vi "Read Status.vi"() -> (0 "Status Data":T1)   [LabVIEW 2012]
doc: "The Basic Serial Read and Write example performs a Serial Port Read, a Serial Port Write, or a combination of these actions. The user selects the actions (read or write) on the front panel. If both are selected, the VI will write the data first, read data, and then close the VISA session that is opened to the port. This VI will wait until the specified number of bytes is received at the port or until a termination character is read.\n\nINSTRUCTIONS:\n1) Select the serial resource and configuration parameters (baud rate, data bits, parity, stop bits, flow control).\n2) Select the operations to be performed. \n3) Connect the serial port to your device. If no device is available, perform a loopback test by doing one of the following. Short pins 2 and 3 on a RS-232 cable or short pin 4 to pin 8 and pin 5 to pin 9 on a RS-485/422 cable. \n4) Run the VI to see the data read. (The \"read string\" will match the \"string to write\" if a loopback test was performed.)\n\nNote: The parameters set for the serial port must match the parameters of the connected instrument or device. In this example, the bytes to read parameter specifies the number of bytes that the serial port reads. If there were more bytes at the port than the number specified in bytes to read, those bytes would not be read. Also, if you specify to read more bytes than the number of bytes actually read, you might receive a timeout error message.\n\nOn the block diagram, the Configure Serial Port VI sets the configuration parameters. The front panel displays the controls used to configure the basic parameters, such as baud rate, data bits, and parity. Constants configure the other parameters the user probably does not need set. After the VISA Configure Serial Port VI opens the VISA session and configures the port, the VI passes the VISA resource name to other VIs that perform operations on that VISA resource. The VISA Write function sends a command to the serial device and the VISA Read function returns data based on the command. The VISA Close function then closes the reference to the serial device. It is important to close the reference; otherwise communication through with that port through protocols other than VISA might not be possible."
uses:
  Correlator port.vi
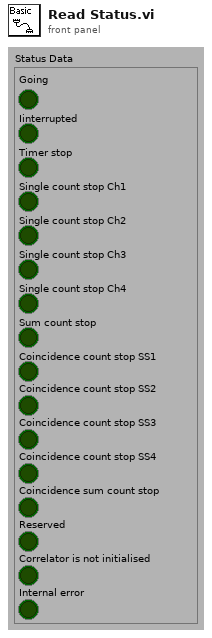
[diagram p1: front panel]
types:
  T1 = cluster{"Going":bool, "Iinterrupted":bool, "Timer stop":bool, "Single count stop Ch1":bool, "Single count stop Ch2":bool, "Single count stop Ch3":bool, "Single count stop Ch4":bool, "Sum count stop":bool, "Coincidence count stop SS1":bool, "Coincidence count stop SS2":bool, "Coincidence count stop SS3":bool, "Coincidence count stop SS4":bool, "Coincidence sum count stop":bool, "Reserved":bool, "Correlator is not initialised":bool, "Internal error":bool}
  T2 = cluster{"unsigned byte array[0]":u8, "unsigned byte array[1]":u8}
  T3 = cluster{"Boolean array[0]":bool, "Boolean array[1]":bool, "Boolean array[2]":bool, "Boolean array[3]":bool, "Boolean array[4]":bool, "Boolean array[5]":bool, "Boolean array[6]":bool, "Boolean array[7]":bool}
  T4 = cluster{"Boolean array[0]":bool, "Boolean array[1]":bool, "Boolean array[2]":bool, "Boolean array[3]":bool, "Boolean array[4]":bool, "Boolean array[5]":bool, "Boolean array[6]":bool, "Boolean array[7]":bool, "Boolean array[0]":bool, "Boolean array[1]":bool, "Boolean array[2]":bool, "Boolean array[3]":bool, "Boolean array[4]":bool, "Boolean array[5]":bool, "Boolean array[6]":bool, "Boolean array[7]":bool}
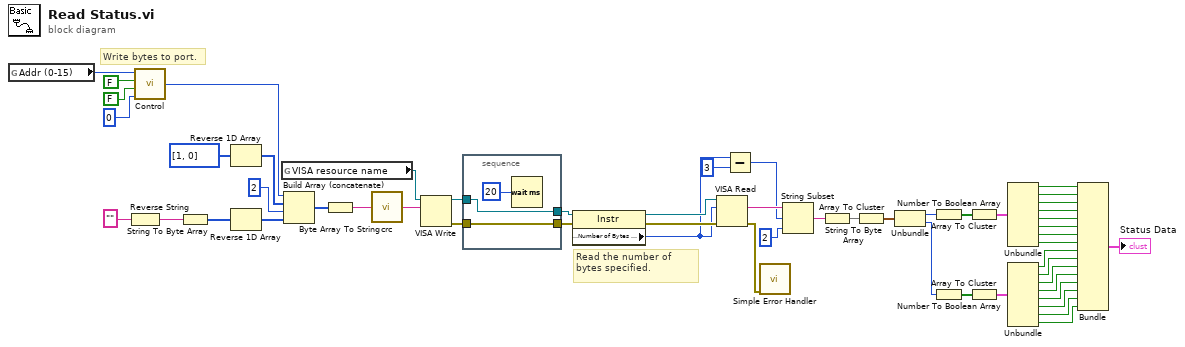
[diagram p0: block diagram]
diagram:
  # "Read the number of bytes specified."
  # "Write bytes to port."
  n1 = global read "Correlator port.vi" "Addr (0-15)"() -> (w7:i8)
  n2 = Reverse String(1:"" ("Data")) -> (0:w9:string)
  n3 = call "Control.vi"("Page"=i8 0, "Error"=FALSE, "Write"=FALSE, "Addr"=w7) -> ("Control Byte"=w19:u32)
  n4 = String To Byte Array(string=w9) -> (unsigned byte array=w14:u8[])
  n5 = Reverse 1D Array(array=i8[] [1, 0] ("Offset")) -> (reversed array=w17:i8[])
  n6 = Reverse 1D Array(array=w14) -> (reversed array=w13:u8[])
  n7 = global read "Correlator port.vi" "VISA resource name"() -> (w8:refnum<visa-resource-name>)
  n8 = Build Array (concatenate)(w19, w17, u8 2 ("Length"), w13) -> (w12:u32[])
  n9 = Byte Array To String(unsigned byte array=w12) -> (string=w11:string)
  n10 = call "crc.vi"("Input string"=w11) -> ("Output (with crc)"=w10:string)
  n11 = VISA Write(VISA resource name=w8, write buffer=w10) -> (VISA resource name out=w52:refnum<visa-resource-name>, error out=w54:errorcluster)  [unwired: 1 in, 1 out]
  n12 = stacked-sequence {
    tunnel: w54 -> [w57]
    tunnel: [w57] -> w53
    tunnel: w52 -> [w56]
    tunnel: [w56] -> w51
    frame #0 {
      n13 = Wait (ms)(milliseconds to wait=u32 20 ("delay before read (ms)")) -> ()  [unwired: 1 out]
    }
  }
  n14 = property class="Instr"(reference=w51, error in=w53) -> (reference out=w5:refnum<visa-resource-name>, error out=w4:errorcluster, "Serial Settings:Number of Bytes at Serial Port"=w3:u32)
  n15 = VISA Read(VISA resource name=w5, byte count=w3, error in (no error)=w4) -> (read buffer=w50:string, error out=w6:errorcluster)  [unwired: 2 out]
  n16 = Subtract(x=w3, y=u32 3) -> (x-y=w1:u32)
  n17 = call <vilib>:"Simple Error Handler.vi"("error in (no error)"=w6) -> ()  [unwired: 1 in, 8 out]
  n18 = String Subset(string=w50, offset (0)=w1, length (rest)=2 ("length (rest)")) -> (substring=w48:string)
  n19 = String To Byte Array(string=w48) -> (unsigned byte array=w47:u8[])
  n20 = Array To Cluster(array=w47) -> (cluster=w46:T2)
  n21 = Unbundle(w46) -> ("unsigned byte array[0]"=w45:u8, "unsigned byte array[1]"=w44:u8)
  n22 = Number To Boolean Array(number=w45) -> (Boolean array=w43:bool[])
  n23 = Number To Boolean Array(number=w44) -> (Boolean array=w42:bool[])
  n24 = Array To Cluster(array=w43) -> (cluster=w41:T3)
  n25 = Array To Cluster(array=w42) -> (cluster=w40:T3)
  n26 = Unbundle(w41) -> ("Boolean array[0]"=w39:bool, "Boolean array[1]"=w38:bool, "Boolean array[2]"=w37:bool, "Boolean array[3]"=w36:bool, "Boolean array[4]"=w35:bool, "Boolean array[5]"=w34:bool, "Boolean array[6]"=w33:bool, "Boolean array[7]"=w32:bool)
  n27 = Unbundle(w40) -> ("Boolean array[0]"=w31:bool, "Boolean array[1]"=w30:bool, "Boolean array[2]"=w29:bool, "Boolean array[3]"=w28:bool, "Boolean array[4]"=w27:bool, "Boolean array[5]"=w26:bool, "Boolean array[6]"=w25:bool, "Boolean array[7]"=w24:bool)
  n28 = Bundle("Boolean array[0]"=w39, "Boolean array[1]"=w38, "Boolean array[2]"=w37, "Boolean array[3]"=w36, "Boolean array[4]"=w35, "Boolean array[5]"=w34, "Boolean array[6]"=w33, "Boolean array[7]"=w32, "Boolean array[0]"=w31, "Boolean array[1]"=w30, "Boolean array[2]"=w29, "Boolean array[3]"=w28, "Boolean array[4]"=w27, "Boolean array[5]"=w26, "Boolean array[6]"=w25, "Boolean array[7]"=w24) -> (→"Status Data":T4)  [unwired: 1 in]
